vi "acqComponentsInit_v3.vi"(1 "sCMOS init":cluster{"init":i16, "sCMOS handle":u32}, 2 "XY stage":T3, 3 "Z stage":T2, 4 "Filter wheel init":cluster{"FW Handle":u32, "init?":i16}, 5 "LSFM_3 lasers":T1(array[cluster])=[{"Component ID"="405nm", "COM Port"="COM14", "Type "=enum."omicronLuxX", "init"=1, "Max power (mW)"=0.0}, {"Component ID"="488nm", "COM Port"="COM4", "Type "=enum."omicronLuxX", "init"=1, "Max power (mW)"=0.0}, {"Component ID"="561nm", "COM Port"="COM27", "Type "=enum."coherentObis", "init"=1, "Max power (mW)"=0.0}, {"Component ID"="642nm", "COM Port"="COM12", "Type "=enum."omicronLuxX", "init"=1, "Max power (mW)"=0.0}], 6 "405 nm (aq)":bool=TRUE, 7 "405 filter":u8(ring)=1 items=["460/36 [DAPI]"=1, "525/50 [FITC]"=2, "605/70 [Cy3]"=3, "665/LP [Cy5]"=4, "Empty-1"=5, "Empty-2"=6], 8 "488 nm (aq)":bool=TRUE, 9 "488 filter":u8(ring)=2 items=["460/36 [DAPI]"=1, "525/50 [FITC]"=2, "605/70 [Cy3]"=3, "665/LP [Cy5]"=4, "Empty-1"=5, "Empty-2"=6], 10 "561 nm (aq)":bool=TRUE, 11 "561 filter":u8(ring)=3 items=["460/36 [DAPI]"=1, "525/50 [FITC]"=2, "605/70 [Cy3]"=3, "665/LP [Cy5]"=4, "Empty-1"=5, "Empty-2"=6], 12 "642 nm (aq)":bool=TRUE, 13 "642 filter":u8(ring)=4 items=["460/36 [DAPI]"=1, "525/50 [FITC]"=2, "605/70 [Cy3]"=3, "665/LP [Cy5]"=4, "Empty-1"=5, "Empty-2"=6]) -> (14 "corrCompsInit?":i16, 15 "noColours":i32, 16 "FWpos":u8[](array[numeric]), 17 "acqLaserCOM":refnum<visa-resource-name>[](array[refnum]), 18 "acqLaserOff":string[](array[string]), 19 "acqLaserOn":string[](array[string]))   [LabVIEW 2015]
panel:
  out "Correct lasers init?":i16=1
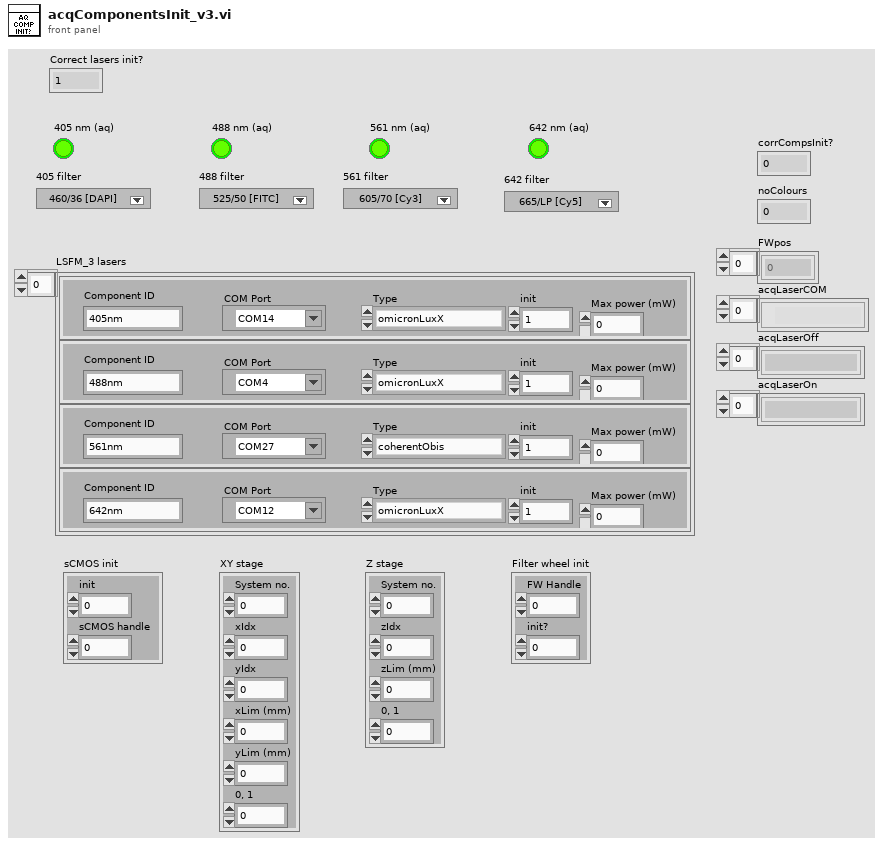
[diagram p1: front panel]
types:
  T1 = cluster{"Component ID":string, "COM Port":refnum<visa-resource-name>, "Type ":enum16{"omicronLuxX", "coherentObis"}, "init":i16, "Max power (mW)":dbl}[]
  T2 = cluster{"System no.":i32, "zIdx":i32, "zLim (mm)":dbl, "0, 1":i16}
  T3 = cluster{"System no.":i32, "xIdx":i32, "yIdx":i32, "xLim (mm)":dbl, "yLim (mm)":dbl, "0, 1":i16}
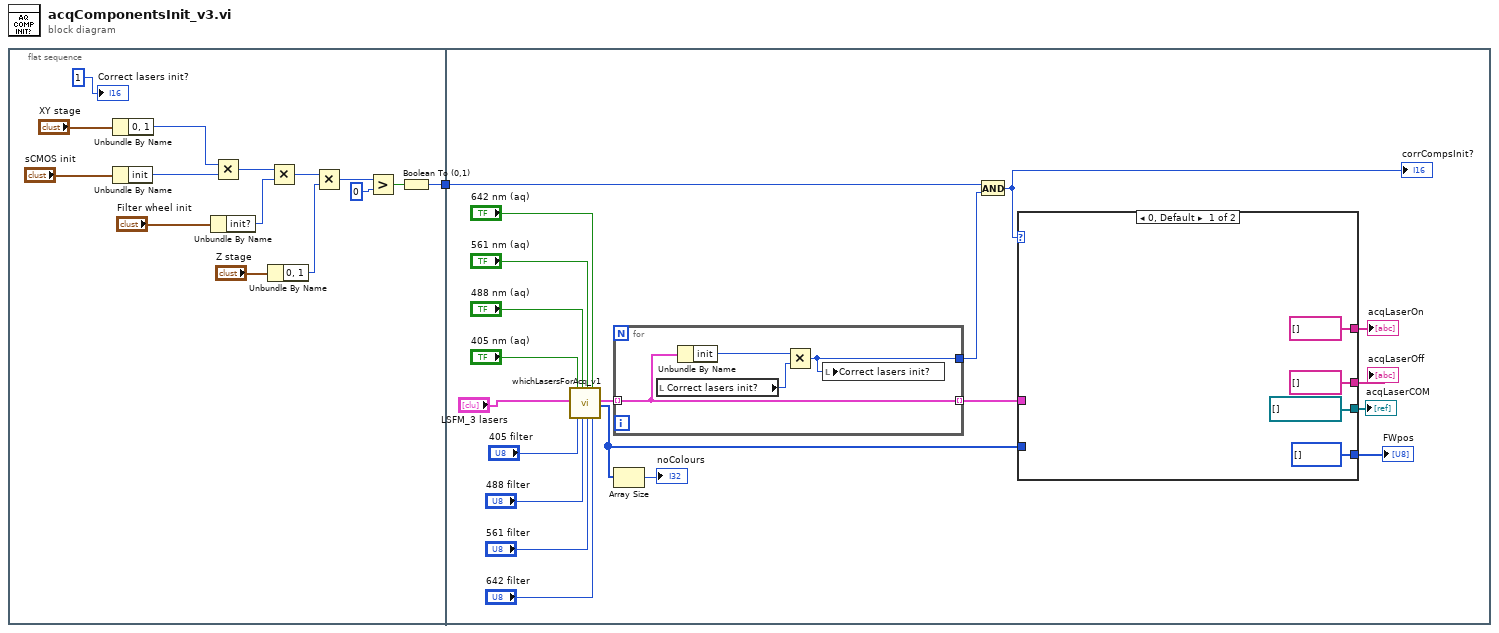
[diagram p0: block diagram]
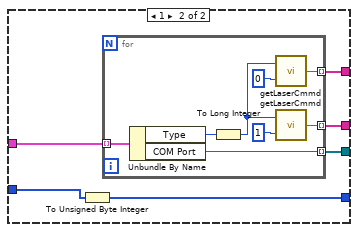
[diagram p2: hidden frame]
diagram:
  n1 = flat-sequence {
    tunnel: [w2] -> w1
    tunnel: w1 -> [w23]
    frame #0 {
      n2 = Unbundle By Name("XY stage") -> ("0, 1"=w12:i16)
      n3 = Unbundle By Name("sCMOS init") -> ("init"=w11:i16)
      n4 = Unbundle By Name("Filter wheel init") -> ("init?"=w9:i16)
      n5 = Multiply(x=w12, y=w11) -> (x*y=w10:i16)
      n6 = Unbundle By Name("Z stage") -> ("0, 1"=w7:i16)
      n7 = Multiply(x=w10, y=w9) -> (x*y=w8:i16)
      n8 = Multiply(x=w8, y=w7) -> (x*y=w6:i16)
      n9 = Greater?(x=w6, y=i16 0) -> (0:w3:bool)
      n10 = Boolean To (0,1)(Boolean=w3) -> (0, 1=w2:i16)
      "Correct lasers init?" <- i16 1 ("Correct lasers init?")
    }
    frame #1 {
      n11 = call "whichLasersForAcq_v1.vi"("LSFM_3 lasers"="LSFM_3 lasers", "405 nm (aq)"="405 nm (aq)", "405 filter"="405 filter", "488 nm (aq)"="488 nm (aq)", "488 filter"="488 filter", "561 nm (aq)"="561 nm (aq)", "561 filter"="561 filter", "642 nm (aq)"="642 nm (aq)", "642 filter"="642 filter") -> ("initLasers"=w28:T1, "initFilters"=w22:u8[])  [unwired: 9 in]
      n12 = for {
        tunnel: w28 -> [w56] mode=indexing
        tunnel: [w57] -> w24
        tunnel: [w56] -> w25 mode=indexing
        n13 = local read "Correct lasers init?"() -> (w58:i16)
        n14 = Unbundle By Name(w56) -> ("init"=w55:i16)
        n15 = Multiply(x=w55, y=w58) -> (x*y=w57:i16)
        n16 = local write "Correct lasers init?"(w57) -> ()
      }
      n17 = Array Size(array=w22) -> (size(s)=→"noColours":i32)
      n18 = And(x=w23, y=w24) -> (x .and. y?=w26:i16)
      "corrCompsInit?" <- w26
      n19 = case shown="0, Default" w26 {
        tunnel: [string[] [] w46] -> w18
        tunnel: [string[] [] w45] -> w19
        tunnel: [refnum<visa-resource-name>[] [] w44] -> w20
        tunnel: w25 -> [_ w43]
        tunnel: w22 -> [_ w42]
        tunnel: [u8[] [] w41] -> w21
        frame 0, Default {
        }
        frame 1 {
          n20 = To Unsigned Byte Integer(number=w42) -> (unsigned 8bit integer=w41:u8[])
          n21 = for {
            tunnel: w43 -> [w54] mode=indexing
            tunnel: [w53] -> w44 mode=indexing
            tunnel: [w48] -> w46 mode=indexing
            tunnel: [w47] -> w45 mode=indexing
            n22 = Unbundle By Name(w54) -> ("Type"=w52:enum16{"omicronLuxX", "coherentObis"}, "COM Port"=w53:refnum<visa-resource-name>)
            n23 = To Long Integer(number=w52) -> (32bit integer=w51:i32)
            n24 = call "getLaserCmmd.vi"("Cmmd index"=0, "Laser type"=w51) -> ("Laser command"=w48:string)
            n25 = call "getLaserCmmd.vi"("Cmmd index"=1, "Laser type"=w51) -> ("Laser command"=w47:string)
          }
        }
      }
      "FWpos" <- w21
      "acqLaserCOM" <- w20
      "acqLaserOff" <- w19
      "acqLaserOn" <- w18
    }
  }
